vi "UT1E3_MaquinaEstados.vi"() -> ()   [LabVIEW 2025]
panel:
  out "Estado Actual":T1(ring)
  out "Delgadas":dbl
  out "Gruesas":dbl
  out "LT":bool
  out "Indicador \nTaladro":dbl(slide)
  out "Taladro Broca":i32(slide)
  out "Pieza":bool
  out "HT":bool
  out "L":bool
  out "H":bool
  in  "SH":bool
  out "a3":bool
  out "a2":bool
  out "a1":bool
  out "a0":bool
  in  "PARO":bool
  in  "START":bool
  in  "stop":bool
  # "sh"
  # "Total de piezas \nterminadas:"
  # "Elaborado por:\n- Bautista Montano Enrique\n- De La Torre Cruz Salma Galilea\n- Sigala Martínez Alejandro"
  # "Pieza en proceso:"
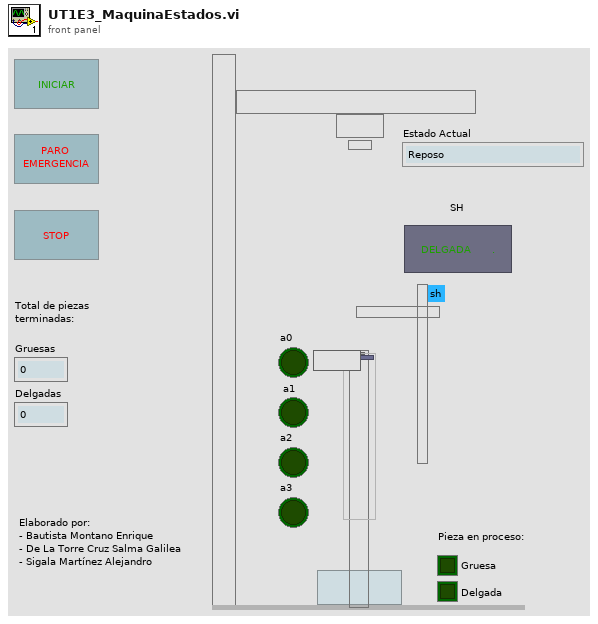
[diagram p1: front panel]
types:
  T1 = enum16{"Reposo", "Avance hasta a1", "Sensar en a1", "Pieza delgada: Avance hasta a3", "Pieza delgada: posición a3", "Pieza delgada: Retorno hasta a2", "Pieza gruesa: Avance hasta a2", "Pieza gruesa: posición a2", "Pieza gruesa: Retorno hasta a1", "Pieza gruesa: Posición a1", "Pieza gruesa: Avance hasta a3", "Pieza gruesa: Posición a3", "Pieza gruesa: Retorno hasta a2", "Posición a2 (tras terminar pieza)", "Retorno hasta a0", "Posición a0 (Inicia nuevo ciclo)"}
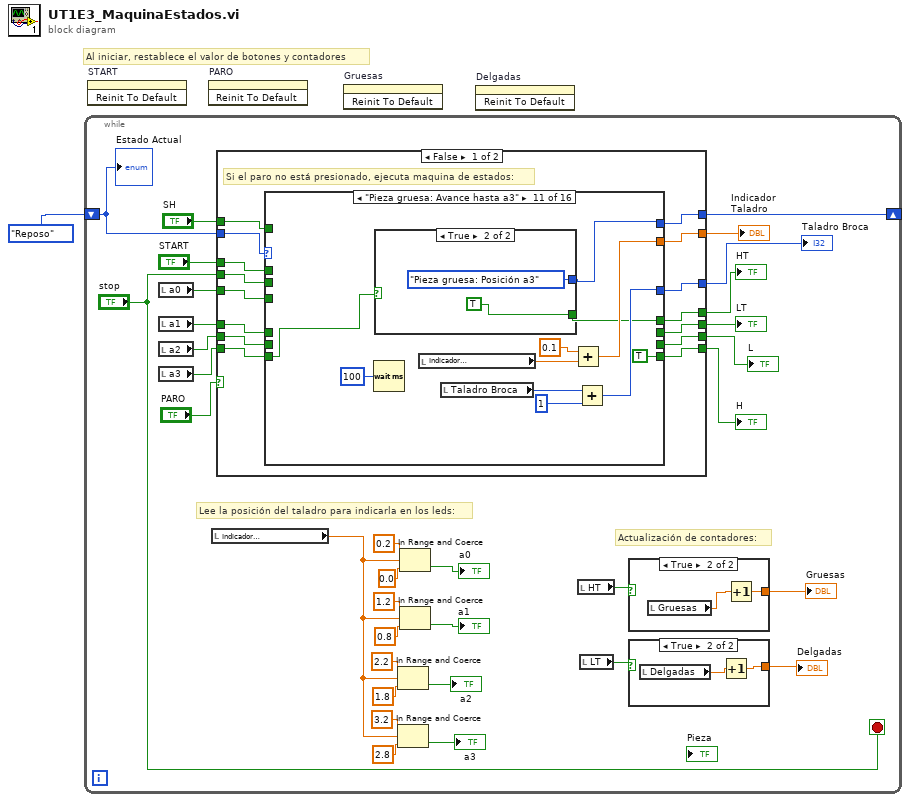
[diagram p0: block diagram]
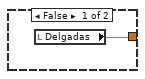
[diagram p2: hidden frame]
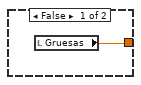
[diagram p3: hidden frame]
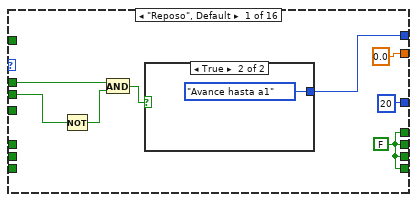
[diagram p4: hidden frame]
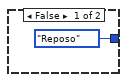
[diagram p5: hidden frame]
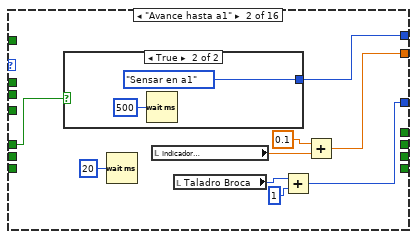
[diagram p6: hidden frame]
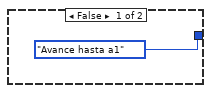
[diagram p7: hidden frame]
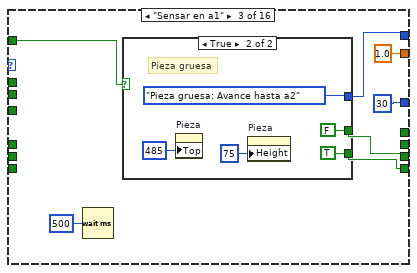
[diagram p8: hidden frame]
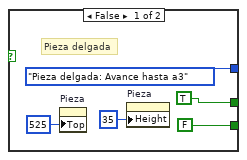
[diagram p9: hidden frame]
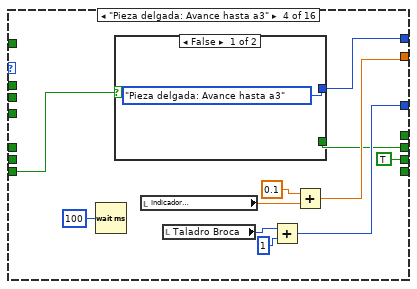
[diagram p10: hidden frame]
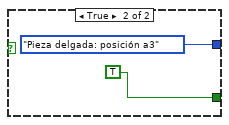
[diagram p11: hidden frame]
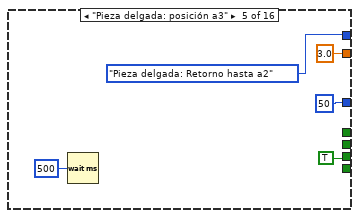
[diagram p12: hidden frame]
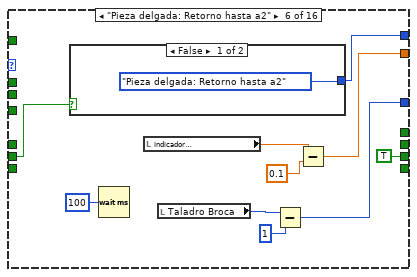
[diagram p13: hidden frame]
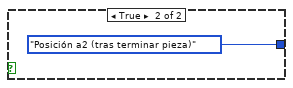
[diagram p14: hidden frame]
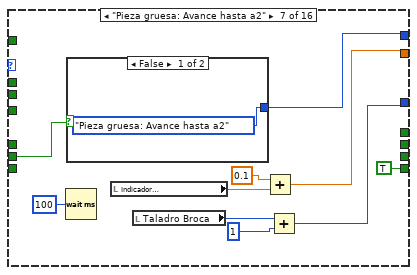
[diagram p15: hidden frame]
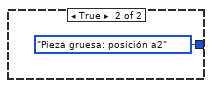
[diagram p16: hidden frame]
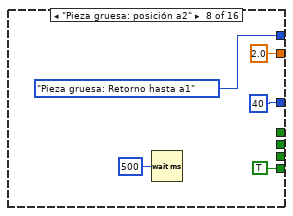
[diagram p17: hidden frame]
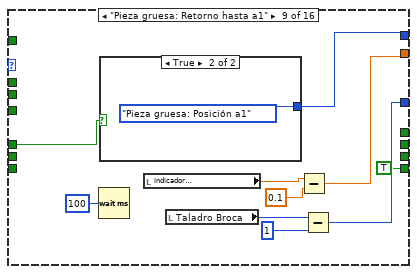
[diagram p18: hidden frame]
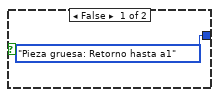
[diagram p19: hidden frame]
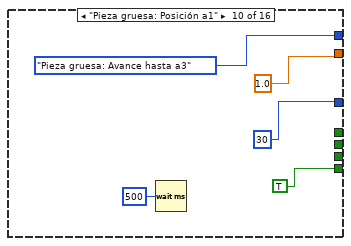
[diagram p20: hidden frame]
diagram:
  # "Al iniciar, restablece el valor de botones y contadores"
  n1 = while {
    shift-right: [w27] -> _
    shift-left: T1."Reposo" -> [w19]
    stop <- "stop" stop-if-true
    # "Actualización de contadores:"
    # "Lee la posición del taladro para indicarla en los leds:"
    n2 = local read "a0"() -> (w30:bool)
    n3 = local read "a1"() -> (w31:bool)
    n4 = local read "a2"() -> (w28:bool)
    n5 = local read "a3"() -> (w29:bool)
    n6 = local read "Indicador \nTaladro"() -> (w8:dbl)
    n7 = case shown="False" "PARO" {
      tunnel: w19 -> [w55 w213]
      tunnel: "START" -> [w54 _]
      tunnel: "SH" -> [w53 _]
      tunnel: "stop" -> [w52 _]
      tunnel: w31 -> [w51 _]
      tunnel: w30 -> [w50 _]
      tunnel: w29 -> [w49 _]
      tunnel: w28 -> [w48 _]
      tunnel: [w47 w213] -> w27
      tunnel: [w46 w215] -> w26
      tunnel: [w45 w214] -> w25
      tunnel: [w44 w219] -> w24
      tunnel: [w43 w216] -> w23
      tunnel: [w42 w218] -> w22
      tunnel: [w41 w217] -> w21
      frame False {
        # "Si el paro no está presionado, ejecuta maquina de estados:"
        n8 = case shown="\"Pieza gruesa: Avance hasta a3\"" w55 {
          tunnel: w54 -> [w63 _ _ _ _ _ _ _ _ _ _ _ _ _ _ w206]
          tunnel: w53 -> [_ _ w83 _ _ _ _ _ _ _ _ _ _ _ _ _]
          tunnel: w52 -> [w62 _ _ _ _ _ _ _ _ _ _ _ _ _ _ _]
          tunnel: [w59 w74 w80 w104 T1."Pieza delgada: Retorno hasta a2" w115 w134 T1."Pieza gruesa: Retorno hasta a1" w148 T1."Pieza gruesa: Avance hasta a3" w164 T1."Pieza gruesa: Retorno hasta a2" w179 T1."Retorno hasta a0" w198 w209] -> w47
          tunnel: [20 w66 30 w98 50 w118 w127 40 w145 30 w162 50 w181 40 w195 20] -> w46
          tunnel: [0.0 w70 1.0 w99 3.0 w117 w128 2.0 w144 1.0 w163 3.0 w182 2.0 w196 0.0] -> w45
          tunnel: [w56 _ w78 _ _ _ TRUE TRUE TRUE TRUE TRUE TRUE TRUE _ _ _] -> w44
          tunnel: [w56 _ w79 TRUE TRUE TRUE _ _ _ _ _ _ _ _ _ _] -> w43
          tunnel: [w56 _ _ _ _ _ _ _ _ _ w160 _ _ _ _ _] -> w42
          tunnel: [w56 _ _ w95 _ _ _ _ _ _ _ _ _ _ _ _] -> w41
          tunnel: w51 -> [_ w73 _ _ _ _ _ _ w149 _ _ _ _ _ _ _]
          tunnel: w50 -> [_ _ _ _ _ _ _ _ _ _ _ _ _ _ w197 _]
          tunnel: w49 -> [_ _ _ w105 _ _ _ _ _ _ w165 _ _ _ _ _]
          tunnel: w48 -> [_ _ _ _ _ w116 w135 _ _ _ _ _ w183 _ _ _]
          frame "Reposo", Default {
            w56 = FALSE
            n9 = Not(x=w62) -> (.not. x?=w61:bool)
            n10 = And(x=w63, y=w61) -> (x .and. y?=w60:bool)
            n11 = case shown="True" w60 {
              tunnel: [T1."Reposo" T1."Avance hasta a1"] -> w59
              frame False {
              }
              frame True {
              }
            }
          }
          frame "Avance hasta a1" {
            n12 = case shown="True" w73 {
              tunnel: [T1."Avance hasta a1" T1."Sensar en a1"] -> w74
              frame False {
              }
              frame True {
                n13 = Wait (ms)(milliseconds to wait=u32 500) -> ()  [unwired: 1 out]
              }
            }
            n14 = Wait (ms)(milliseconds to wait=u32 20) -> ()  [unwired: 1 out]
            n15 = local read "Indicador \nTaladro"() -> (w69:dbl)
            n16 = local read "Taladro Broca"() -> (w68:i32)
            n17 = Add(x=w68, y=1) -> (x+y=w66:i32)
            n18 = Add(x=0.1, y=w69) -> (x+y=w70:dbl)
          }
          frame "Sensar en a1" {
            n19 = Wait (ms)(milliseconds to wait=u32 500) -> ()  [unwired: 1 out]
            n20 = case shown="True" w83 {
              tunnel: [T1."Pieza delgada: Avance hasta a3" T1."Pieza gruesa: Avance hasta a2"] -> w80
              tunnel: [TRUE FALSE] -> w79
              tunnel: [FALSE TRUE] -> w78
              frame False {
                # "Pieza delgada"
                n21 = property on="Pieza" class="Bool"("Top"=525 ("Position:Top")) -> ()  [unwired: 2 in, 2 out]
                n22 = property on="Pieza" class="Bool"("Height"=u32 35 ("Button Size:Height")) -> ()  [unwired: 2 in, 2 out]
              }
              frame True {
                # "Pieza gruesa"
                n23 = property on="Pieza" class="Bool"("Top"=485 ("Position:Top")) -> ()  [unwired: 2 in, 2 out]
                n24 = property on="Pieza" class="Bool"("Height"=u32 75 ("Button Size:Height")) -> ()  [unwired: 2 in, 2 out]
              }
            }
          }
          frame "Pieza delgada: Avance hasta a3" {
            n25 = Wait (ms)(milliseconds to wait=u32 100) -> ()  [unwired: 1 out]
            n26 = case shown="False" w105 {
              tunnel: [T1."Pieza delgada: Avance hasta a3" T1."Pieza delgada: posición a3"] -> w104
              tunnel: [_ TRUE] -> w95
              frame False {
              }
              frame True {
              }
            }
            n27 = local read "Indicador \nTaladro"() -> (w101:dbl)
            n28 = local read "Taladro Broca"() -> (w100:i32)
            n29 = Add(x=w100, y=1) -> (x+y=w98:i32)
            n30 = Add(x=0.1, y=w101) -> (x+y=w99:dbl)
          }
          frame "Pieza delgada: posición a3" {
            n31 = Wait (ms)(milliseconds to wait=u32 500) -> ()  [unwired: 1 out]
          }
          frame "Pieza delgada: Retorno hasta a2" {
            n32 = case shown="False" w116 {
              tunnel: [T1."Pieza delgada: Retorno hasta a2" T1."Posición a2 (tras terminar pieza)"] -> w115
              frame False {
              }
              frame True {
              }
            }
            n33 = Wait (ms)(milliseconds to wait=u32 100) -> ()  [unwired: 1 out]
            n34 = local read "Indicador \nTaladro"() -> (w120:dbl)
            n35 = local read "Taladro Broca"() -> (w122:i32)
            n36 = Subtract(x=w122, y=1) -> (x-y=w118:i32)
            n37 = Subtract(x=w120, y=0.1 ("x")) -> (x-y=w117:dbl)
          }
          frame "Pieza gruesa: Avance hasta a2" {
            n38 = Wait (ms)(milliseconds to wait=u32 100) -> ()  [unwired: 1 out]
            n39 = case shown="False" w135 {
              tunnel: [T1."Pieza gruesa: Avance hasta a2" T1."Pieza gruesa: posición a2"] -> w134
              frame False {
              }
              frame True {
              }
            }
            n40 = local read "Indicador \nTaladro"() -> (w131:dbl)
            n41 = local read "Taladro Broca"() -> (w130:i32)
            n42 = Add(x=0.1, y=w131) -> (x+y=w128:dbl)
            n43 = Add(x=w130, y=1) -> (x+y=w127:i32)
          }
          frame "Pieza gruesa: posición a2" {
            n44 = Wait (ms)(milliseconds to wait=u32 500) -> ()  [unwired: 1 out]
          }
          frame "Pieza gruesa: Retorno hasta a1" {
            n45 = Wait (ms)(milliseconds to wait=u32 100) -> ()  [unwired: 1 out]
            n46 = case shown="True" w149 {
              tunnel: [T1."Pieza gruesa: Retorno hasta a1" T1."Pieza gruesa: Posición a1"] -> w148
              frame False {
              }
              frame True {
              }
            }
            n47 = local read "Indicador \nTaladro"() -> (w146:dbl)
            n48 = local read "Taladro Broca"() -> (w152:i32)
            n49 = Subtract(x=w146, y=0.1 ("x")) -> (x-y=w144:dbl)
            n50 = Subtract(x=w152, y=1) -> (x-y=w145:i32)
          }
          frame "Pieza gruesa: Posición a1" {
            n51 = Wait (ms)(milliseconds to wait=u32 500) -> ()  [unwired: 1 out]
          }
          frame "Pieza gruesa: Avance hasta a3" {
            n52 = Wait (ms)(milliseconds to wait=u32 100) -> ()  [unwired: 1 out]
            n53 = case shown="True" w165 {
              tunnel: [T1."Pieza gruesa: Avance hasta a3" T1."Pieza gruesa: Posición a3"] -> w164
              tunnel: [_ TRUE] -> w160
              frame False {
              }
              frame True {
              }
            }
            n54 = local read "Indicador \nTaladro"() -> (w170:dbl)
            n55 = local read "Taladro Broca"() -> (w169:i32)
            n56 = Add(x=0.1, y=w170) -> (x+y=w163:dbl)
            n57 = Add(x=w169, y=1) -> (x+y=w162:i32)
          }
          frame "Pieza gruesa: Posición a3" {
            n58 = Wait (ms)(milliseconds to wait=u32 500) -> ()  [unwired: 1 out]
          }
          frame "Pieza gruesa: Retorno hasta a2" {
            n59 = Wait (ms)(milliseconds to wait=u32 100) -> ()  [unwired: 1 out]
            n60 = case shown="True" w183 {
              tunnel: [T1."Pieza gruesa: Retorno hasta a2" T1."Posición a2 (tras terminar pieza)"] -> w179
              frame False {
              }
              frame True {
              }
            }
            n61 = local read "Indicador \nTaladro"() -> (w184:dbl)
            n62 = local read "Taladro Broca"() -> (w188:i32)
            n63 = Subtract(x=w184, y=0.1 ("x")) -> (x-y=w182:dbl)
            n64 = Subtract(x=w188, y=1) -> (x-y=w181:i32)
          }
          frame "Posición a2 (tras terminar pieza)" {
            n65 = Wait (ms)(milliseconds to wait=u32 500) -> ()  [unwired: 1 out]
          }
          frame "Retorno hasta a0" {
            n66 = Wait (ms)(milliseconds to wait=u32 20) -> ()  [unwired: 1 out]
            n67 = case shown="True" w197 {
              tunnel: [T1."Retorno hasta a0" T1."Posición a0 (Inicia nuevo ciclo)"] -> w198
              frame False {
              }
              frame True {
              }
            }
            n68 = local read "Indicador \nTaladro"() -> (w202:dbl)
            n69 = local read "Taladro Broca"() -> (w203:i32)
            n70 = Subtract(x=w202, y=0.1 ("x")) -> (x-y=w196:dbl)
            n71 = Subtract(x=w203, y=1) -> (x-y=w195:i32)
          }
          frame "Posición a0 (Inicia nuevo ciclo)" {
            n72 = case shown="False" w206 {
              tunnel: [T1."Reposo" T1."Avance hasta a1"] -> w209
              frame False {
              }
              frame True {
              }
            }
            n73 = Wait (ms)(milliseconds to wait=u32 500) -> ()  [unwired: 1 out]
          }
        }
      }
      frame True {
        # "Paro de emergencia presionado:\nMáquina de estados en pausa, actuadores detenidos."
        n74 = local read "Taladro Broca"() -> (w215:i32)
        n75 = local read "Indicador \nTaladro"() -> (w214:dbl)
        n76 = local read "HT"() -> (w218:bool)
        n77 = local read "LT"() -> (w217:bool)
        n78 = local read "L"() -> (w216:bool)
        n79 = local read "H"() -> (w219:bool)
      }
    }
    "Indicador \nTaladro" <- w25
    "Taladro Broca" <- w26
    "H" <- w24
    "L" <- w23
    "HT" <- w22
    "LT" <- w21
    n80 = In Range and Coerce(upper limit=2.2, x=w8, lower limit=1.8) -> (In Range?=→"a2":bool)  [unwired: 1 out]
    n81 = In Range and Coerce(upper limit=3.2, x=w8, lower limit=2.8) -> (In Range?=→"a3":bool)  [unwired: 1 out]
    n82 = In Range and Coerce(upper limit=0.2, x=w8, lower limit=0.0) -> (In Range?=→"a0":bool)  [unwired: 1 out]
    n83 = In Range and Coerce(upper limit=1.2, x=w8, lower limit=0.8) -> (In Range?=→"a1":bool)  [unwired: 1 out]
    n84 = local read "HT"() -> (w5:bool)
    n85 = local read "LT"() -> (w3:bool)
    n86 = case shown="True" w5 {
      tunnel: [w38 w39] -> w4
      frame False {
        n87 = local read "Gruesas"() -> (w38:dbl)
      }
      frame True {
        n88 = local read "Gruesas"() -> (w40:dbl)
        n89 = Increment(x=w40) -> (x+1=w39:dbl)
      }
    }
    "Gruesas" <- w4
    n90 = case shown="True" w3 {
      tunnel: [w35 w36] -> w2
      frame False {
        n91 = local read "Delgadas"() -> (w35:dbl)
      }
      frame True {
        n92 = local read "Delgadas"() -> (w37:dbl)
        n93 = Increment(x=w37) -> (x+1=w36:dbl)
      }
    }
    "Delgadas" <- w2
    "Estado Actual" <- w19
  }
  n94 = invoke on="START" class="Bool (strict)" method="Reinit To Default"() -> ()  [unwired: 3 in, 3 out]
  n95 = invoke on="PARO" class="Bool (strict)" method="Reinit To Default"() -> ()  [unwired: 3 in, 3 out]
  n96 = invoke on="Gruesas" class="DigNum (strict)" method="Reinit To Default"() -> ()  [unwired: 3 in, 3 out]
  n97 = invoke on="Delgadas" class="DigNum (strict)" method="Reinit To Default"() -> ()  [unwired: 3 in, 3 out]
